vi "Example tcp data collector events.vi"() -> ()   [LabVIEW 2020]
uses:
  TCP subscription info cluster.ctl
  MySQL/Preset Query Enum.ctl
panel:
  out "All data":string[][](array[string])
  out "device times all data received":cluster{"Device":string, "time":u32}[](array[cluster])
  out "dev times timeout":cluster{"Device":string, "time":u32}[](array[cluster])
  out "time waited":u32(graph)
  out "timeout":bool
  out "time":u32 caption="time waiting"
  in  "timeout for get all devs (ms)":u32=5000
  out "Devs no data":string[](array[string])
  in  "Device/Devicetype name\n/Plotter.id/#":string
  out "timeout":bool
  out "loop time":u32
  out "Device name":string
  out "TCP subscriptions info":T1
  in  "stop":bool
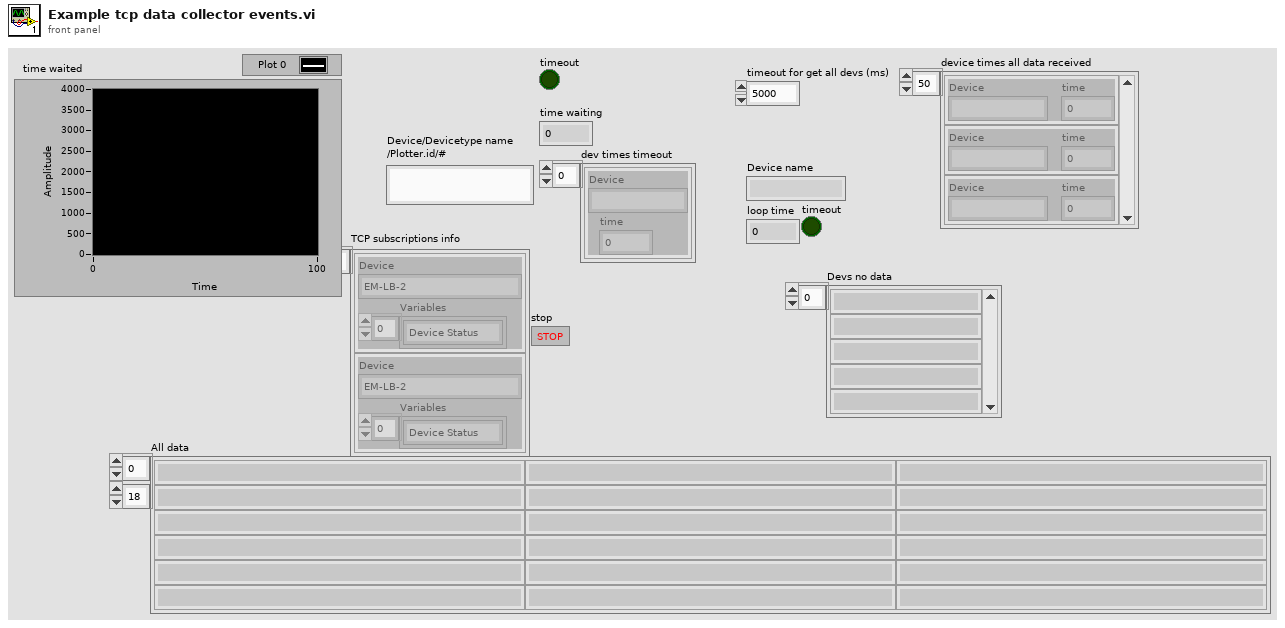
[diagram p1: front panel]
types:
  T1 = typedef "TCP subscription info cluster.ctl" = cluster{"Device":string, "Variables":string[]}[]
  T2 = typedef "Preset Query Enum.ctl" = enum16{"Get Locations", "Get all IPs and MACs", "Get classes", "Get expt variables to set at scanstart for particular device", "Get expt devices and variables with start values", "Get expt devices and variables (with data to get)", "Get expt devices with data to get", "Get Expt devices and GUIs", "Get all devices basic properties", "Get Virtual Devices Core Info", "Get Expt names", "Get experiment basic properties", "Get experiment alarm variables", "Get MC Ports", "Get device network comm port", "Get devicetype lvclass path", "Get basic device properties", "Get Init Order", "Get all setable variables of a device", "Get device variable aliases", "Get force values of all settable variables", "Get all variables of a devicetype", "Get all variables of a device", "Get plotter details", "Get Saved Scans", "Get Scan Info", "GetGeneralGUIs", "Get expt for plotter", "Get plotter IDs from expt", "Get all devices", "Get all Virtual Devices", "Get all aliases", "Get variable and device info for Virtual Device", "GetItemLocatorIP", "Get IPs for GUIs", "Get DeviceType from Device", "GetLocalPortRange", "GetDevicePresetVariables", "Get Device Configuration", "GetAllPresetNames", "GetAllConfigurationNames", "GetPresetDeviceNames", "GetDeviceAliases", "GetDevicesOfClass"}
  T3 = typedef "tcp_new_data_event.ctl" = refnum<user-event>
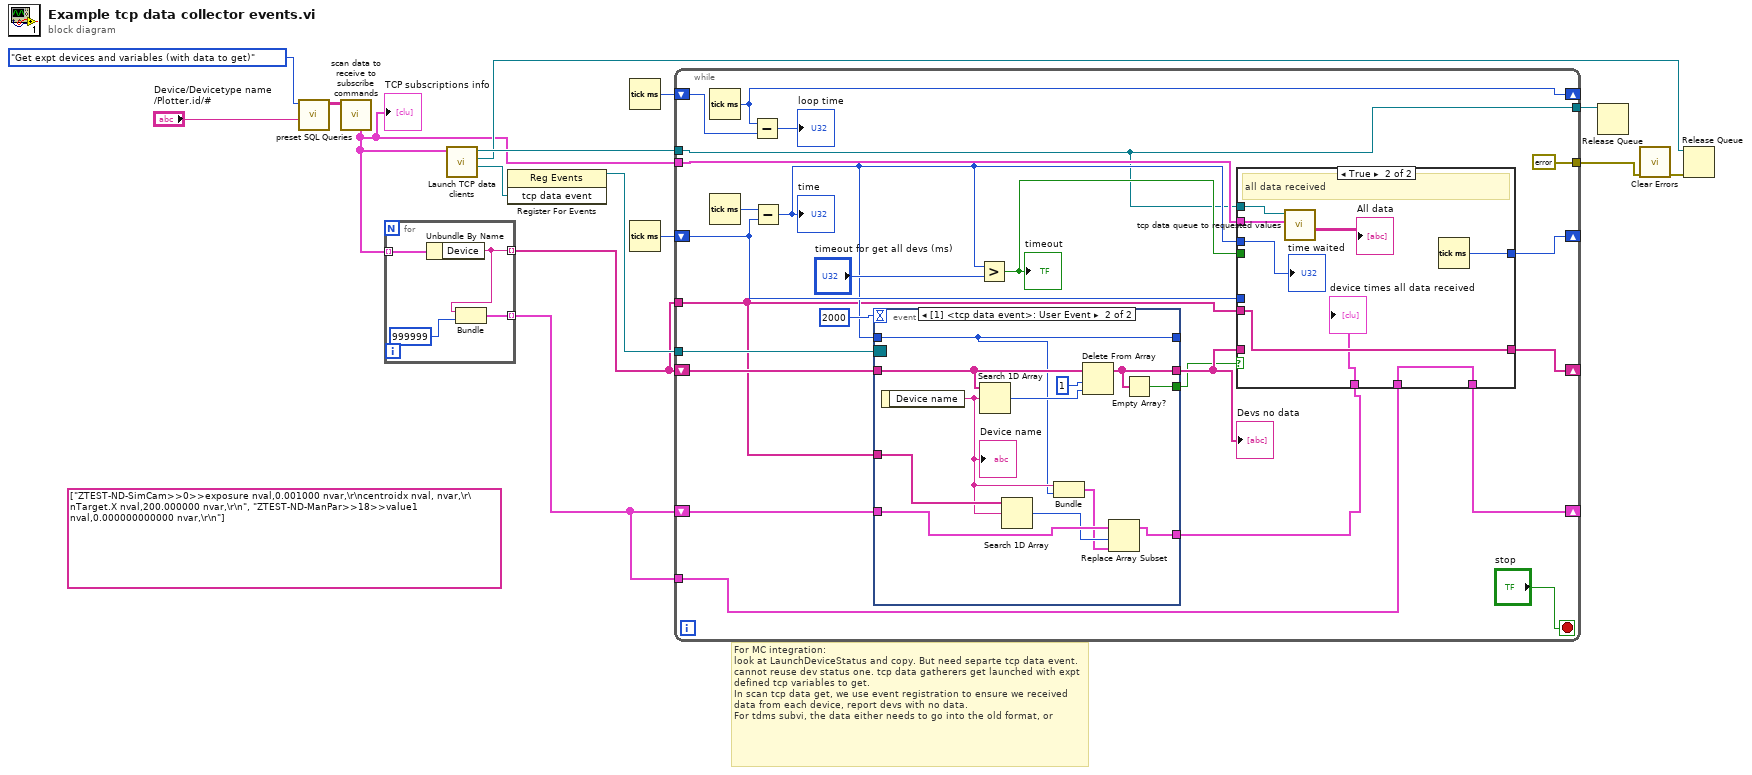
[diagram p0: block diagram]
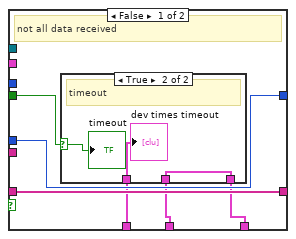
[diagram p2: hidden frame]
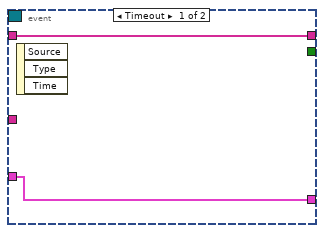
[diagram p4: hidden frame]
diagram:
  (unwired) string[] ["ZTEST-ND-SimCam>>0>>exposure nval,0.001000 nvar,\r\ncentroidx nval, nvar,\r\nTarget.X nval,200.000000 nvar,\r\n", "ZTEST-ND-ManPar>>18>>value1 nval,0.000000000000 nvar,\r\n"] ("Scan data in")
  # "For MC integration:\nlook at LaunchDeviceStatus and copy. But need separte tcp data event. cannot reuse dev status one. tcp data gatherers get launched with expt defined tcp variables to get.\nIn scan tcp data get, we use event registration to ensure we received data from each device, report devs with no data.\nFor tdms subvi, the data either needs to go into the old format, or"
  n1 = call "preset SQL Queries.vi"("Expt name / MCIP/ Variable/Preset Name"="Device/Devicetype name\n/Plotter.id/#", "Preset Query"=Preset_Query_Enum."Get expt devices and variables (with data to get)") -> ("data"=w6:string[][])  [unwired: 7 in, 2 out]
  n2 = call "scan data to receive to subscribe commands.vi"("ScanData to receive"=w6) -> ("TCP subscriptions info"=w5:T1)  [unwired: 7 in, 3 out]
  "TCP subscriptions info" <- w5
  n3 = for {
    tunnel: w5 -> [w19] mode=indexing
    tunnel: [w18] -> w4 mode=indexing
    tunnel: [w16] -> w2 mode=indexing
    n4 = Unbundle By Name(w19) -> ("Device"=w18:string)
    n5 = Bundle("Device"=w18, "time"=u32 999999) -> (w16:cluster{"Device":string, "time":u32})  [unwired: 1 in]
  }
  n6 = call "Launch TCP data clients.vi"("TCP subscriptions info"=w5) -> ("tcp data event"=w11:T3, "StopQueue"=w13:refnum<queue>, "DataQueue"=w15:refnum<queue>)  [unwired: 8 in]
  n7 = register-events(w11) -> (reference out=w10:refnum<event-registration>)  [unwired: 2 in, 1 out]
  n8 = Tick Count (ms)() -> (millisecond timer value=w9:u32)
  n9 = Tick Count (ms)() -> (millisecond timer value=w3:u32)
  n10 = while {
    tunnel: w15 -> [w21]
    tunnel: [w21] -> w14
    tunnel: w5 -> [w22]
    tunnel: w10 -> [w42]
    shift-right: [w40] -> _
    shift-left: w9 -> [w39]
    shift-right: [w30] -> _
    shift-left: w4 -> [w37]
    tunnel: w4 -> [w28]
    shift-right: [w34] -> _
    shift-left: w3 -> [w33]
    shift-right: [w24] -> _
    shift-left: w2 -> [w27]
    tunnel: w2 -> [w25]
    tunnel: [errorcluster {"status"=FALSE, "code"=0, "source"=""} ("error in (no error)")] -> w1
    stop <- "stop" stop-if-true
    n11 = Tick Count (ms)() -> (millisecond timer value=w40:u32)
    n12 = Tick Count (ms)() -> (millisecond timer value=w36:u32)
    n13 = Subtract(x=w40, y=w39) -> (x-y=→"loop time":u32)
    n14 = Subtract(x=w36, y=w33) -> (x-y=w29:u32)
    "time" <- w29
    n15 = event shown="[1] <tcp data event>: User Event" {
      selector: w42 -> [_ _]
      dyn-events: _ -> [_ _]
      timeout: 2000 -> [_ _]
      tunnel: w37 -> [w63 w73]
      tunnel: [w63 w72] -> w31
      tunnel: [_ w71] -> w23
      tunnel: [_ w66] -> _
      tunnel: w29 -> [_ w66]
      tunnel: w28 -> [_ w70]
      tunnel: w27 -> [w62 w69]
      tunnel: [w62 w64] -> w26
      event Timeout {
        n16 = event-data() -> ()  [unwired: 1 in, 3 out]
      }
      event User Event {
        n17 = event-data() -> ("Device name"=w68:string)  [unwired: 1 in]
        "Device name" <- w68
        n18 = Search 1D Array(1D array=w73, element=w68) -> (index of element=w75:i32)  [unwired: 1 in]
        n19 = Search 1D Array(1D array=w70, element=w68) -> (index of element=w67:i32)  [unwired: 1 in]
        n20 = Bundle("Device name"=w68, w66) -> (w65:cluster{"Device name":string, u32})  [unwired: 1 in]
        n21 = Delete From Array(array=w73, length=1, index=w75) -> (array with subset deleted=w72:string[])  [unwired: 1 out]
        n22 = Replace Array Subset(array=w69, new element=w65, index=w67) -> (w64:cluster{"Device":string, "time":u32}[])
        n23 = Empty Array?(array=w72) -> (empty?=w71:bool)
      }
    }
    "Devs no data" <- w31
    n24 = Greater?(x=w29, y="timeout for get all devs (ms)") -> (0:w32:bool)
    "timeout" <- w32
    n25 = case shown="True" w23 {
      tunnel: [w49 w61] -> w34
      tunnel: w33 -> [w49 _]
      tunnel: w32 -> [w48 _]
      tunnel: w28 -> [_ w60]
      tunnel: w31 -> [w47 _]
      tunnel: [w47 w60] -> w30
      tunnel: w29 -> [_ w59]
      tunnel: w26 -> [w46 w58]
      tunnel: w25 -> [w44 w57]
      tunnel: [w45 w57] -> w24
      tunnel: w22 -> [_ w56]
      tunnel: w21 -> [_ w55]
      frame False {
        # "not all data received"
        n26 = case shown="True" w48 {
          selector: w48 -> [_ w51]
          tunnel: w46 -> [w50 w53]
          tunnel: [w50 w52] -> w45
          tunnel: w44 -> [_ w52]
          frame False {
            # "not timed out yet"
          }
          frame True {
            # "timeout"
            "dev times timeout" <- w53
            "timeout" <- w51
          }
        }
      }
      frame True {
        # "all data received"
        n27 = call "tcp data queue to requested values.vi"("TCP subscriptions info"=w56, "Queue in"=w55) -> ("All data"=→"All data":string[][])  [unwired: 6 in, 3 out]
        n28 = Tick Count (ms)() -> (millisecond timer value=w61:u32)
        "time waited" <- w59
        "device times all data received" <- w58
      }
    }
  }
  n29 = Release Queue(queue=w14) -> ()  [unwired: 2 in, 3 out]
  n30 = call <vilib>:"Clear Errors.vi"("error in (no error)"=w1) -> ("error out"=w12:errorcluster)  [unwired: 5 in, 1 out]
  n31 = Release Queue(queue=w13, error in (no error)=w12) -> ()  [unwired: 1 in, 3 out]
